vi "Test Sim Fill FIFO.vi"() -> ()   [LabVIEW 2013]
uses:
  <vilib>/rvi/interface/common/niFpgaWaitOnOcc.vi
  <vilib>/Utility/error.llb/Error Cluster From Error Code.vi
  <vilib>/rvi/errors/niLvFpgaAdjustHostInterfaceError.vi
  <vilib>/rvi/interface/nirviMethod/nirviMethod.xnode
  Host/FGs/FPGA_Reference.ctl
  FPGA Bitfiles/WingBeatAnalyzer_FPGATargetSim_10_2.lvbitx
  10-Tap 8-bit Camera without DRAM (FPGA-SIM).vi
  <vilib>/rvi/interface/nirviReadWriteControl/nirviReadWriteControl.xnode
  <vilib>/FPGAPlugInAG/PCIe-7842R/niLvFpga_WriteFifo_PCIe-7842R.vi
  <vilib>/rvi/errors/niLvFpgaMergeErrorWithErrorCode.vi
  NiFpgaLv.dll
panel:
  out "Words per image":u32
  out "Target Sim TO":bool
  out "Empty Elements Remaining":u32
  in  "stop":bool
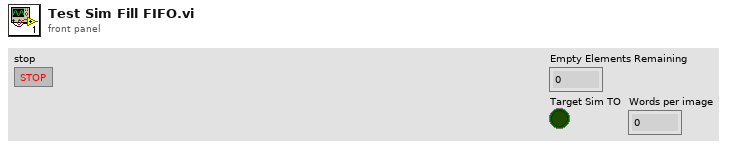
[diagram p1: front panel]
types:
  T1 = typedef "FPGA_Reference.ctl" = refnum<k20>
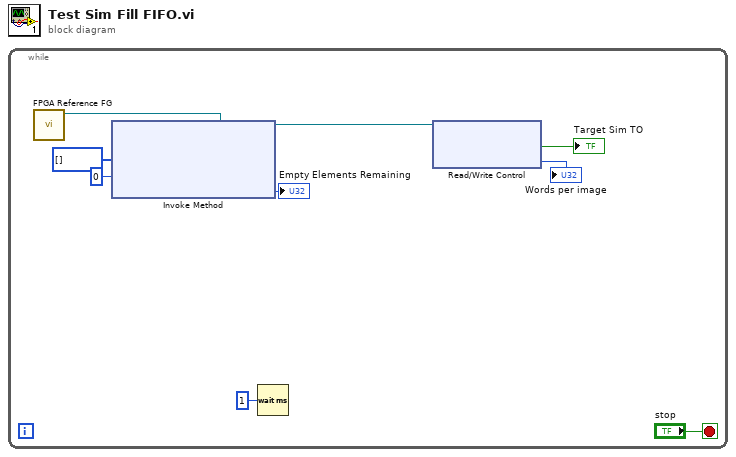
[diagram p0: block diagram]
diagram:
  n1 = while {
    stop <- "stop" stop-if-true
    n2 = call "FPGA Reference FG.vi"() -> ("FPGA VI Reference Out"=w9:T1)  [unwired: 11 in]
    n3 = xnode "Invoke Method"("FPGA VI Reference In"=w9, "Data"=u64[] [], "Timeout (ms)"=0) -> ("FPGA VI Reference Out"=w3:T1, "Empty Elements Remaining"=→"Empty Elements Remaining":u32)  [unwired: 1 in, 1 out]
    n4 = Wait (ms)(milliseconds to wait=u32 1) -> ()  [unwired: 1 out]
    n5 = xnode "Read/Write Control"("FPGA VI Reference In"=w3) -> ("Target Sim TO"=→"Target Sim TO":bool, "Words per image"=→"Words per image":u32)  [unwired: 1 in, 2 out]
  }
